vi "Get Instrument Addon Name.vi"(8 "error in (no error)":errorcluster, 11 "instrument addon refnum in":T1 format="%.0x") -> (0 "error out":errorcluster, 2 "name":string, 3 "instrument addon refnum out":T1=18446744073709551615 format="%.0x")   [LabVIEW 2020, in "Instrument Addon Scripting API.lvlib"]
doc: "Returns the name of an Instrument Addon Custom Device."
uses:
  Instrument Addon Scripting API.lvlib
  <vilib>/NI VeriStand/Custom Device API/Custom Device Item Ref.ctl
  <vilib>/Utility/error.llb/Error Cluster From Error Code.vi
  <vilib>/ErrorRing/Error Ring.xnode
  Dependencies.llb/Instrument_Addon_Scripting_Dependencies_Advanced System Definition.lvlib
  <vilib>/NI VeriStand/Custom Device API/Custom Device API.lvlib
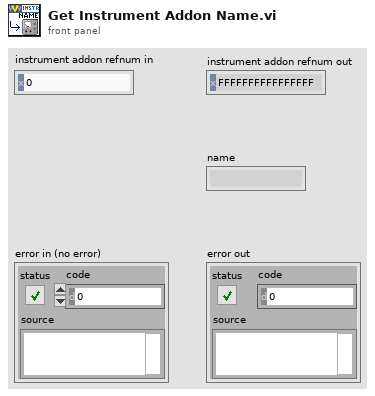
[diagram p1: front panel]
types:
  T1 = typedef "Custom Device API.lvlib/Custom Device Item Ref.ctl" = u64
  T2 = typedef "Instrument_Addon_Scripting_Dependencies_Advanced System Definition.lvlib/Instrument_Addon_Scripting_Dependencies_TreeItem.Info.ctl" = cluster{"Name":string, "Description":string, "GUID":string, "Is Channel":bool, "Channel":T3, "Is Waveform":bool, "Waveform":T5}
  T3 = typedef "Custom Device API.lvlib/Custom Device Channel.ctl" = cluster{"Type":T4, "Units":string, "Default Value":dbl, "Faultable":bool, "Scalable":bool}
  T4 = typedef "Custom Device API.lvlib/Custom Device Channel Type.ctl" = enum16{"Input", "Output"}
  T5 = typedef "Custom Device API.lvlib/Custom Device Waveform.ctl" = cluster{"Data Type":T6, "Units":string}
  T6 = typedef "Custom Device API.lvlib/Custom Device Waveform DataType.ctl" = enum16{"Double", "Complex Double"}
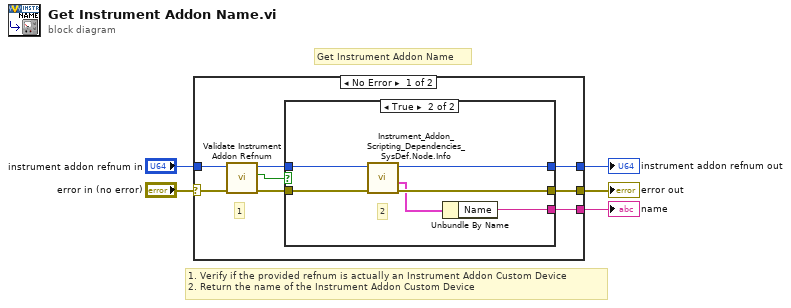
[diagram p0: block diagram]
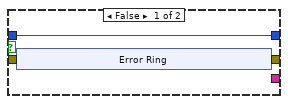
[diagram p2: hidden frame]
diagram:
  # "1. Verify if the provided refnum is actually an Instrument Addon Custom Device\n2. Return the name of the Instrument Addon Custom Device"
  # "Get Instrument Addon Name"
  n1 = case shown="No Error" "error in (no error)" {
    selector: "error in (no error)" -> [w9 w28]
    tunnel: "instrument addon refnum in" -> [w10 w27]
    tunnel: [w13 w28] -> w4
    tunnel: [w12 w27] -> w2
    tunnel: [w11 _] -> w1
    frame No Error {
      # "1"
      n2 = call "Validate Instrument Addon Refnum.vi"("Error In"=w9, "Refnum In"=w10) -> ("Error Out"=w8:errorcluster, "Is Instrument Addon?"=w6:bool, "Refnum Out"=w7:T1)  [unwired: 7 in]
      n3 = case shown="True" w6 {
        tunnel: w7 -> [w14 w26]
        tunnel: [w15 w25] -> w13
        tunnel: [w14 w24] -> w12
        tunnel: [_ w22] -> w11
        tunnel: w8 -> [_ w21]
        frame False {
          n4 = xnode "Error Ring"() -> ("error out"=w15:errorcluster)
        }
        frame True {
          # "2"
          n5 = call "Instrument_Addon_Scripting_Dependencies_SysDef.Node.Info.vi"("error in (no error)"=w21, "nodeID"=w26) -> ("error out"=w25:errorcluster, "Item Info"=w23:T2, "nodeID out"=w24:u64)  [unwired: 6 in, 1 out]
          n6 = Unbundle By Name(w23) -> ("Name"=w22:string)
        }
      }
    }
    frame Error {
    }
  }
  "error out" <- w4
  "instrument addon refnum out" <- w2
  "name" <- w1
